vi "After Launch Init Core.vi"(8 "error in (no error)":errorcluster, 11 "LS218 in":refnum<class "LS218.lvclass">) -> (0 "error out":errorcluster, 3 "LS218 out":refnum<class "LS218.lvclass">)   [LabVIEW 2015, in "LS218.lvlib" / "LS218.lvclass"]
doc: "Use <b>Pre Launch init.vi</b> method for sanity checks that are supposed to prevent the actor from launching if they fail. Use <B>this</B> method instead to initialize this actor when it has been activated. A corresponding high priority message will become dispatched before the <B>Actor Core.vi</b> is called.\n\n<b>Derived classed should call the parent methode first</b> and their own initialization code after.\n\nRefer also to the ongoing discussion at https://decibel.ni.com/content/message/57394#57394."
uses:
  LS218.lvclass
  LS218 Messages/Read All Sensor Data Msg/Read All Sensor Data Msg.lvclass
  LS218 Messages/Read All Sensor Data Msg/Read All Sensor Data Msg.lvclass/Read All Sensor Data Msg.ctl
  LS218.lvclass/LS218.ctl
  <vilib>/ActorFramework/Actor/Actor.lvclass/Actor.ctl
  <vilib>/ActorFramework/Message Enqueuer/Message Enqueuer.lvclass/Message Enqueuer.ctl
  CSPP_Core/Actors/CS++BaseActor/CS++BaseActor.lvclass/CS++BaseActor.ctl
  LS218 Messages/Write calibration curves to instruments Msg/Write calibration curves to instruments Msg.lvclass/Write calibration curves to instruments Msg.ctl
  <vilib>/ActorFramework/Message Enqueuer/Init from Existing Queue.vi
  <vilib>/ActorFramework/Message Enqueuer/Enqueue.vi
  <vilib>/ActorFramework/Message Priority Queue/Priority Enqueue.vi
  <vilib>/ActorFramework/Message Enqueuer/Message Enqueuer.lvclass
  LS218 Messages/Write calibration curves to instruments Msg/Write calibration curves to instruments Msg.lvclass
  CSPP_Core/Actors/CS++DeviceActor/CS++DeviceActor.lvclass
  <vilib>/ActorFramework/Actor/Actor.lvclass
  CSPP_Core/Classes/CS++ProcessVariables/PVConnection/PVConnection.lvclass
  CSPP_Core/Actors/CS++BaseActor/CS++BaseActor.lvclass
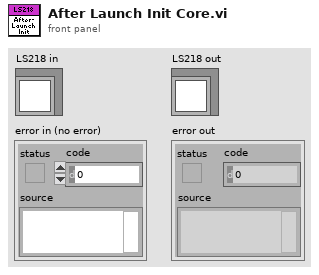
[diagram p1: front panel]
types:
  T1 = cluster{"Write Access":enum8{"Allowed", "Required", "None"}, "Read Access":enum8{"Allowed", "Required", "None"}}
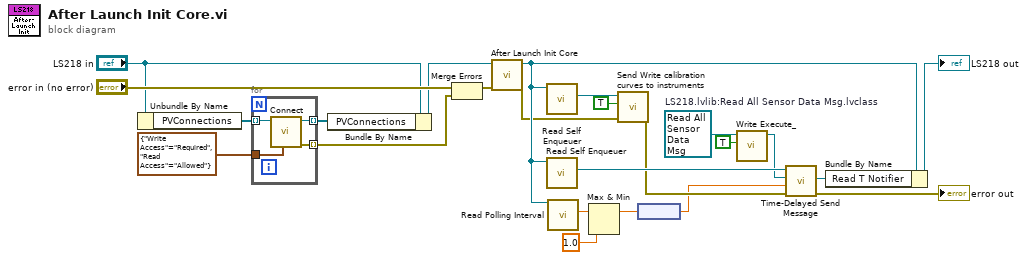
[diagram p0: block diagram]
diagram:
  w2 = refnum<class "Read All Sensor Data Msg.lvclass"> refnum  # LS218.lvlib:Read All Sensor Data Msg.lvclass
  n1 = Unbundle By Name("LS218 in") -> ("PVConnections"=w22:refnum<class "PVConnection.lvclass">[])
  n2 = for {
    tunnel: w22 -> [w28] mode=indexing
    tunnel: [w27] -> w21 mode=indexing
    tunnel: T1 {"Write Access"=enum."Required", "Read Access"=enum."Allowed"} ("Access") -> [w26]
    tunnel: [w25] -> w16 mode=indexing
    n3 = call "Connect.vi"("Access (R/W allowed)"=w26, "PVConnection in"=w28) -> ("Error Out"=w25:errorcluster, "PVConnection out"=w27:refnum<class "PVConnection.lvclass">)  [unwired: 8 in]
  }
  n4 = Bundle By Name(cluster="LS218 in", "PVConnections"=w21) -> (w18:refnum<class "LS218.lvclass">)
  n5 = Merge Errors("error in (no error)", w16) -> (w17:errorcluster)
  n6 = call-parent "After Launch Init Core.vi"("error in (no error)"=w17, "CS++DeviceActor in"=w18) -> ("error out"=w5:errorcluster, "CS++DeviceActor out"=w6:refnum<class "LS218.lvclass">)  [unwired: 8 in]
  n7 = call <vilib>:"Read Self Enqueuer.vi"("Actor"=w6) -> ("Self Enqueuer"=w23:refnum<class "Message Enqueuer.lvclass">)  [unwired: 10 in]
  n8 = call <vilib>:"Read Self Enqueuer.vi"("Actor"=w6) -> ("Self Enqueuer"=w15:refnum<class "Message Enqueuer.lvclass">)  [unwired: 10 in]
  n9 = call "Read Polling Interval.vi"("CS++BaseActor in"=w6) -> ("Polling Interval"=w10:dbl[unit])  [unwired: 8 in, 2 out]
  n10 = Max & Min(x=w10, y=dbl[unit] 1.0) -> (max(x,y)=w8:dbl[unit])  [unwired: 1 out]
  n11 = call "Send Write calibration curves to instruments.vi"("error in (no error)"=w5, "Execute?"=TRUE, "Message Enqueuer"=w23) -> ("error out"=w14:errorcluster)  [unwired: 7 in, 1 out]
  n12 = node(w8) -> (w9:dbl)
  n13 = call "Write Execute_.vi"("Execute?"=TRUE, "Read All Sensor Data Msg in"=w2) -> ("Read All Sensor Data Msg out"=w1:refnum<class "Read All Sensor Data Msg.lvclass">)  [unwired: 8 in, 1 out]
  n14 = call <vilib>:"Time-Delayed Send Message.vi"("error in (no error)"=w14, "Milliseconds To Wait"=w9, "Message"=w1, "Message Enqueuer"=w15) -> ("error out"=→"error out":errorcluster, "Delivery Notifier"=w11:refnum<notifier>)  [unwired: 6 in]
  n15 = Bundle By Name(cluster=w6, "Read T Notifier"=w11) -> (→"LS218 out":refnum<class "LS218.lvclass">)
